vi "Push_Multi_Wrapping_Less.vi"   [LabVIEW 2024, in "POTCircularBuffer.Tests.Units.lvlib"]
uses:
  POTCircularBuffer.Tests.Units.lvlib
  <vilib>/addons/_JKI Toolkits/Caraya/classes/Test/Test.lvclass
  <vilib>/addons/_JKI Toolkits/Caraya/classes/Assert/Assert.lvclass
  <vilib>/addons/_JKI Toolkits/Caraya/classes/Assert/Assert Equal Value_Variant.vi
  Type.ctl
  POTTypedCircularBuffer.lvclass
types:
  T1 = typedef "POTTypedCircularBuffer.lvclass/Type.ctl" = i32
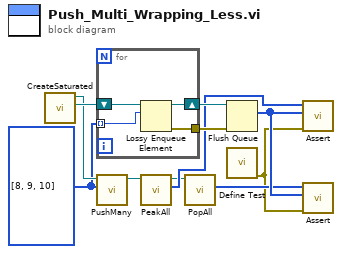
[diagram p0: block diagram]
diagram:
  w6 = T1[] [8, 9, 10] ("Elements")
  n1 = call "CreateSaturated.vi"() -> ("Golden"=w8:refnum<queue>, "POTTypedCircularBuffer out"=w7:refnum<class "POTTypedCircularBuffer.lvclass">)  [unwired: 10 in]
  n2 = for {
    tunnel: [w15] -> w10
    shift-right: [w14] -> w9
    shift-left: w8 -> [w13]
    tunnel: w6 -> [w12] mode=indexing
    n3 = Lossy Enqueue Element(queue=w13, element=w12) -> (queue out=w14:refnum<queue>, error out=w15:errorcluster)  [unwired: 1 in, 2 out]
  }
  n4 = call "PushMany.vi"("Elements"=w6, "POTTypedCircularBuffer in"=w7) -> ("POTTypedCircularBuffer out"=w11:refnum<class "POTTypedCircularBuffer.lvclass">)  [unwired: 9 in]
  n5 = call "PeakAll.vi"("POTTypedCircularBuffer in"=w11) -> ("Copied Buffer"=w5:T1[], "POTTypedCircularBuffer out"=w4:refnum<class "POTTypedCircularBuffer.lvclass">)  [unwired: 9 in]
  n6 = call "PopAll.vi"("POTTypedCircularBuffer in"=w4) -> ("Flushed Buffer"=w2:T1[])  [unwired: 9 in, 1 out]
  n7 = Flush Queue(queue=w9, error in (no error)=w10) -> (remaining elements=w3:T1[])  [unwired: 2 out]
  n8 = call <vilib>:"Define Test.vi"() -> ("error out"=w1:errorcluster)  [unwired: 10 in, 1 out]
  n9 = call-poly <vilib>:"Assert.vi"("error in (no error)"=w1, "Y"=w3, "X"=w5) -> ()  [unwired: 7 in, 2 out]
  n10 = call-poly <vilib>:"Assert.vi"("error in (no error)"=w1, "Y"=w3, "X"=w2) -> ()  [unwired: 7 in, 2 out]
